vi "RS232 DTR RTS.vi"(8 "error in (no error)":errorcluster, 9 "Func":T1(ring), 10 "On/Off":bool=TRUE, 11 "TesterCOM in":refnum<visa-resource-name>="COM3") -> (0 "error out":errorcluster)   [LabVIEW 2017]
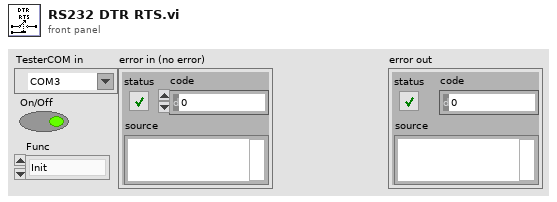
[diagram p1: front panel]
types:
  T1 = enum16{"Init", "VEnable", "PowerOnOff", "PowerONVEnable"}
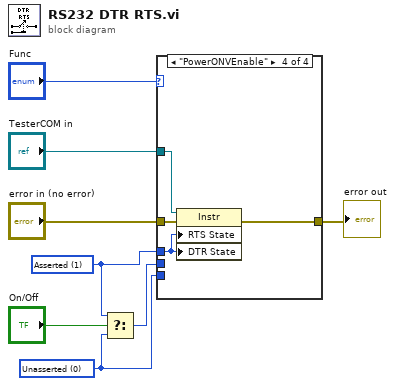
[diagram p0: block diagram]
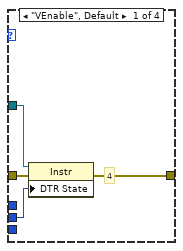
[diagram p2: hidden frame]
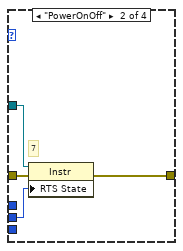
[diagram p3: hidden frame]
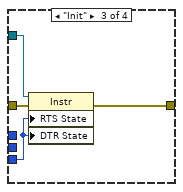
[diagram p4: hidden frame]
diagram:
  w2 = i16 0 items=["Unknown"=-1, "Unasserted"=0, "Asserted"=1] ("Serial Settings:Modem Line Settings:Line RTS State")
  w1 = i16 1 items=["Unknown"=-1, "Unasserted"=0, "Asserted"=1] ("Serial Settings:Modem Line Settings:Line RTS State")
  n1 = Select(t=w1, s="On/Off", f=w2) -> (s? t:f=w5:i16)
  n2 = case shown="\"PowerONVEnable\"" "Func" {
    tunnel: "TesterCOM in" -> [w12 w15 w19 w23]
    tunnel: w5 -> [w11 w16 _ _]
    tunnel: "error in (no error)" -> [w10 w14 w18 w22]
    tunnel: [w9 w13 w20 w24] -> w3
    tunnel: w2 -> [_ _ w17 _]
    tunnel: w1 -> [_ _ _ w21]
    frame "VEnable", Default {
      # "4"
      n3 = property class="Instr"(reference=w12, error in=w10, "DTR State"=w11) -> (error out=w9:errorcluster)  [unwired: 1 out]
    }
    frame "PowerOnOff" {
      # "7"
      n4 = property class="Instr"(reference=w15, error in=w14, "RTS State"=w16) -> (error out=w13:errorcluster)  [unwired: 1 out]
    }
    frame "Init" {
      n5 = property class="Instr"(reference=w19, error in=w18, "RTS State"=w17, "DTR State"=w17) -> (error out=w20:errorcluster)  [unwired: 1 out]
    }
    frame "PowerONVEnable" {
      n6 = property class="Instr"(reference=w23, error in=w22, "RTS State"=w21, "DTR State"=w21) -> (error out=w24:errorcluster)  [unwired: 1 out]
    }
  }
  "error out" <- w3
